vi "GSI-HVSwitch2.get channel voltage.vi"(0 "i ref in":refnum<vi>, 2 "channel":i32, 3 "ms timeout (10000)":i32=10000, 5 "error in (no error)":errorcluster) -> (14 "i ref out":refnum<vi>, 16 "ActVoltage":dbl format="%.2f", 17 "timed out":bool, 19 "error out":errorcluster)   [LabVIEW 2014, in "GSI-HVSwitch2.lvlib"]
doc: "Reads the actual voltage of the instrument."
uses:
  GSI-HVSwitch2.lvlib
  CSCore/CSApplicationBaseClasses/PSChannelBase/PSChannelBase.directionType.ctl
  CSCore/CSApplicationBaseClasses/PSChannelBase/PSChannelBase.serviceType.ctl
  CSlibraries/UtilityLib/UtilityLib.valueStatus.ctl
  CSCore/CSApplicationBaseClasses/DeviceBase/DeviceBase.deviceState.ctl
  CSCore/CSSystem/CoreDefs/CoreDefs.error_type.ctl
  CSCore/CSSystem/CoreDefs/CoreDefs.error_severity.ctl
  CSCore/CSSystem/CoreLib/CoreLib.lvlib
  CSCore/CSApplicationBaseClasses/PSChannelBase/PSChannelBase.lvlib
  CSlibraries/UtilityLib/UtilityLib.lvlib
  CSCore/CSApplicationBaseClasses/DeviceBase/DeviceBase.lvlib
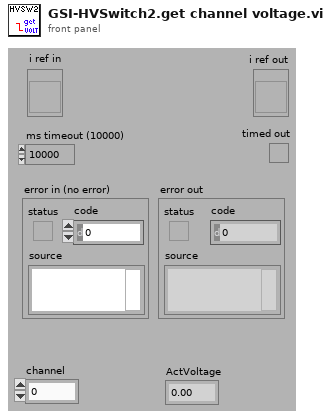
[diagram p1: front panel]
types:
  T1 = typedef "UtilityLib.lvlib/UtilityLib.valueStatus.ctl" = enum16{"no info available", "stand by/off", "on", "warning", "alarm/malfunction", "not implemented", "user action required", "important information", "system default", "control default", "indicator default", "button default"}
  T2 = typedef "PSChannelBase.lvlib/PSChannelBase.serviceType.ctl" = enum16{"onOff", "voltage", "current", "tripCurrent", "rampUpSpeed", "rampDownSpeed", "status"}
  T3 = typedef "PSChannelBase.lvlib/PSChannelBase.directionType.ctl" = enum16{"unknown", "update actual value", "update nominal value", "update both"}
  T4 = typedef "CoreDefs.error_severity.ctl" = enum16{"undefined", "information", "warning", "error", "fatal"}
  T5 = typedef "CoreDefs.error_type.ctl" = enum16{"no error", "can't load process", "can't unload process", "process does not exist", "can't install process", "can't remove process", "unknown function", "time out", "can't execute function", "duplicate queue name", "super not found", "caller queue invalid", "can't ping process", "unknown error", "VISA Error", "VISA timeout", "GPIB timeout", "GPIB error", "communication error", "data type mismatch", "can't read data from OPC server", "can't write data to OPC server", "OET error", "function not implemented", "process already exists", "invalid Shared Variable name", "error writing Shared Variable", "error reading Shared Variable", "invalid client name", "corrupt database", "unknown class", "call not authorized", "parameter out of range", "OET timeout: can't get data to modify", "invalid queue name", "requested operation incompatible with current state", "event undefined", "event disabled", "state undefined", "caller is not a friend", "EventBuilder: bad eventID", "EventBuilder: no DAQ devices", "a thread must not stop itself", "UNUSED ELEMENT4", "DiscArchiver: eventData incomplete", "DiscArchiver: eventData does not belong to run", "DiscArchiver: can't open file", "DiscArchiver: can't write to file", "DiscArchiver: available disc space low", "can't acquire semaphore", "error reading data from database", "notifier object is not existing", "can't register process", "can't unregister process", "illegal event type", "object disabled", "object already exists", "can't change state", "Instrument not found", "no connection to remote node", "invalid reference", "N/A", "UNUSED ELEMENT 1", "element not found", "illegal TCP/IP connection detected", "object does not exist", "invalid access ID", "unknown CS system", "invalid privilige", "unsupported data type", "unsupported server type", "IO server already exists", "Shared Variable already exists"}
  T6 = typedef "DeviceBase.lvlib/DeviceBase.deviceState.ctl" = i16
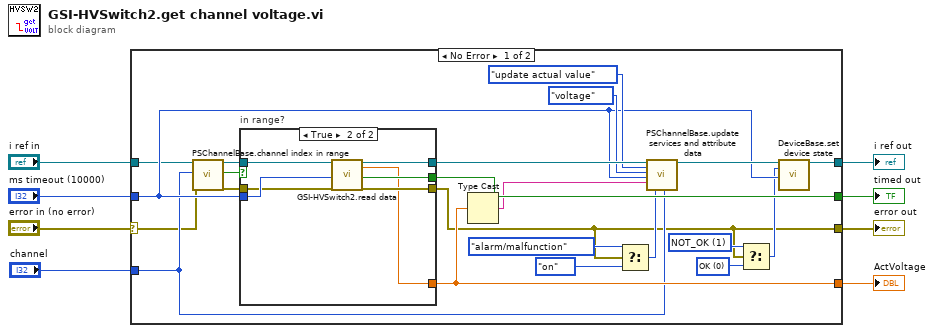
[diagram p0: block diagram]
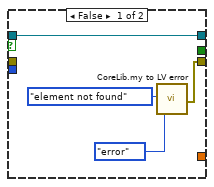
[diagram p2: hidden frame]
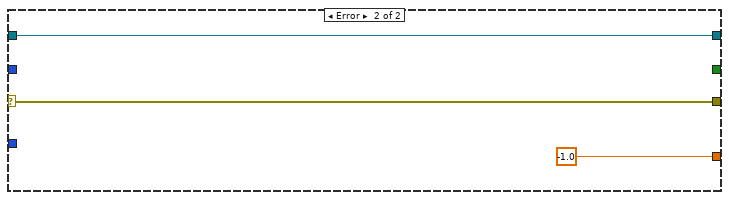
[diagram p3: hidden frame]
diagram:
  n1 = case shown="No Error" "error in (no error)" {
    selector: "error in (no error)" -> [w11 w43]
    tunnel: "i ref in" -> [w15 w44]
    tunnel: "ms timeout (10000)" -> [w19 _]
    tunnel: [w30 _] -> w6
    tunnel: [w20 w44] -> w5
    tunnel: [w9 w43] -> w4
    tunnel: [w26 -1.0 ("ActVoltage")] -> w3
    tunnel: "channel" -> [w13 _]
    frame No Error {
      w17 = T6 1 items=["ERROR"=-1, "OK"=0, "NOT_OK"=1] ("deviceState")
      w18 = T6 0 items=["ERROR"=-1, "OK"=0, "NOT_OK"=1] ("deviceState")
      n2 = call "PSChannelBase.channel index in range.vi"("i ref in"=w15, "channelIndex"=w13, "error in (no error)"=w11) -> ("i ref out"=w14:refnum<vi>, "in range"=w12:bool, "error out"=w10:errorcluster)  [unwired: 14 in]
      n3 = case "in range?" shown="True" w12 {
        tunnel: w14 -> [w32 w41]
        tunnel: w19 -> [_ w40]
        tunnel: [_ w39] -> w30
        tunnel: [w32 w35] -> w29
        tunnel: [w31 w38] -> w9
        tunnel: [_ w37] -> w26
        tunnel: w10 -> [_ w36]
        frame False {
          n4 = call "CoreLib.my to LV error.vi"("ErrorTypes"=CoreDefs.error_type."element not found", "severityLevel"=CoreDefs.error_severity."error") -> ("myErrorCluster"=w31:errorcluster)  [unwired: 16 in, 1 out]
        }
        frame True {
          n5 = call "GSI-HVSwitch2.read data.vi"("i ref in"=w41, "ms timeout (10000)"=w40, "error in (no error)"=w36) -> ("i ref out"=w35:refnum<vi>, "ActVoltage"=w37:dbl, "timed out"=w39:bool, "error out"=w38:errorcluster)  [unwired: 10 in, 3 out]
        }
      }
      n6 = Type Cast(x=w26) -> (*(type *) &x=w25:string)  [unwired: 1 in]
      n7 = Select(t=UtilityLib.valueStatus."alarm/malfunction" ("quality"), s=w9, f=UtilityLib.valueStatus."on") -> (s? t:f=w22:T1)
      n8 = call "PSChannelBase.update services and attribute data.vi"("i ref in"=w29, "direction"=PSChannelBase.directionType."update actual value", "service"=PSChannelBase.serviceType."voltage", "ms timeout (10000)"=w19, "value"=w25, "quality"=w22, "channelNumber"=w13) -> ("i ref out"=w21:refnum<vi>)  [unwired: 10 in, 2 out]
      n9 = Select(t=w17, s=w9, f=w18) -> (s? t:f=w16:T6)
      n10 = call "DeviceBase.set device state.vi"("i ref in"=w21, "deviceState"=w16, "ms timeout (10000)"=w19) -> ("i ref out"=w20:refnum<vi>)  [unwired: 14 in, 2 out]
    }
    frame Error {
    }
  }
  "error out" <- w4
  "i ref out" <- w5
  "timed out" <- w6
  "ActVoltage" <- w3
